vi "Get Voltage.vi"(8 "error in (no error)":errorcluster, 10 "Voltage":dbl, 11 "APG in":refnum<class "APG.lvclass">) -> (0 "error out":errorcluster, 3 "APG out":refnum<class "APG.lvclass">)   [LabVIEW 2021, in "APG.lvlib" / "APG.lvclass"]
uses:
  APG.lvclass
  APG.lvclass/APG.ctl
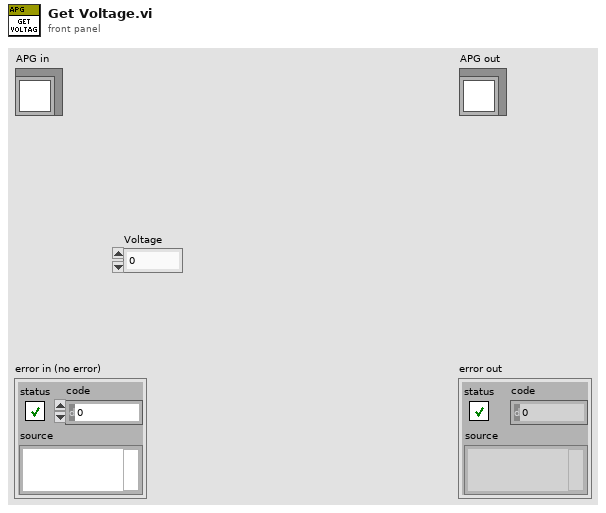
[diagram p1: front panel]
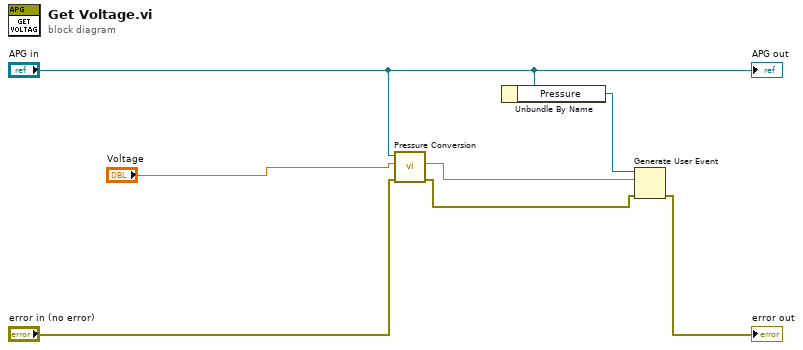
[diagram p0: block diagram]
diagram:
  n1 = call "Pressure Conversion.vi"("error in (no error)"="error in (no error)", "Voltage"="Voltage", "APG in"="APG in") -> ("error out"=w2:errorcluster, "Pressure"=w3:dbl)  [unwired: 7 in]
  n2 = Unbundle By Name("APG in") -> ("Pressure"=w4:refnum<user-event>)
  n3 = Generate User Event(user event=w4, event data cluster=w3, error in=w2) -> (error out=→"error out":errorcluster)  [unwired: 1 in, 1 out]
  "APG out" <- "APG in"
